vi "First LV Actor Launcher.vi"   [LabVIEW 2020, in "First LV Actor.lvlib"]
uses:
  First LV Actor.lvlib
  Demo Actor/Demo Actor.lvclass
  C:/Program Files (x86)/National Instruments/LabVIEW 2020/vi.lib/ActorFramework/Actor/Actor.lvclass
  <vilib>/ActorFramework/Actor/Actor.lvclass
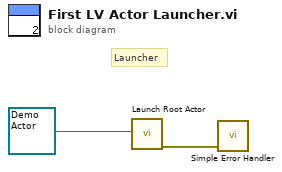
[diagram p0: block diagram]
diagram:
  # "Launcher"
  n1 = call <vilib>:"Launch Root Actor.vi"("Actor"=refnum<class "Demo Actor.lvclass"> refnum ("First LV Actor.lvlib:Demo Actor.lvclass")) -> ("error out"=w1:errorcluster)  [unwired: 9 in, 1 out]
  n2 = call <vilib>:"Simple Error Handler.vi"("error in (no error)"=w1) -> ()  [unwired: 4 in, 5 out]
